vi "Write Return DER_Measurement Msg.vi"(10 "Return DER_Measurement Msg":refnum<class "Return DER_Measurement Msg.lvclass">, 11 "EMS Generic in":refnum<class "EMS Generic.lvclass">) -> (3 "EMS Generic out":refnum<class "EMS Generic.lvclass">)   [LabVIEW 2018, in "EMS Generic Actor.lvlib" / "EMS Generic.lvclass"]
uses:
  EMS Generic.lvclass
  EMS Generic Messages/Return DER_Measurement Msg/Return DER_Measurement Msg.lvclass
  EMS Generic.lvclass/EMS Generic.ctl
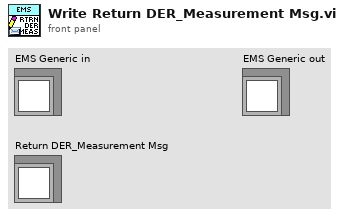
[diagram p1: front panel]
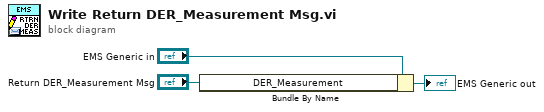
[diagram p0: block diagram]
diagram:
  n1 = Bundle By Name(cluster="EMS Generic in", "DER_Measurement"="Return DER_Measurement Msg") -> (→"EMS Generic out":refnum<class "EMS Generic.lvclass">)
